vi "notification_option.vi"(11 "your_email":string) -> (1 "pick_up_code":string, 2 "go_to_the_address":string, 3 "to_receive":string)   [LabVIEW 2023]
uses:
  <vilib>/Utility/file.llb/Read Delimited Spreadsheet (string).vi
  Global 1.vi
panel:
  out "substring":string
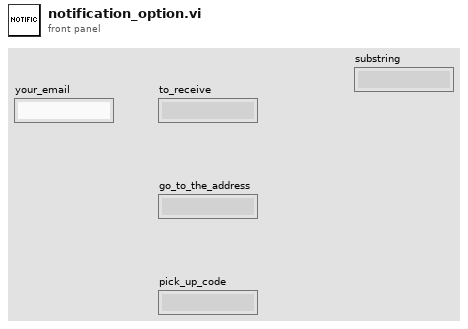
[diagram p1: front panel]
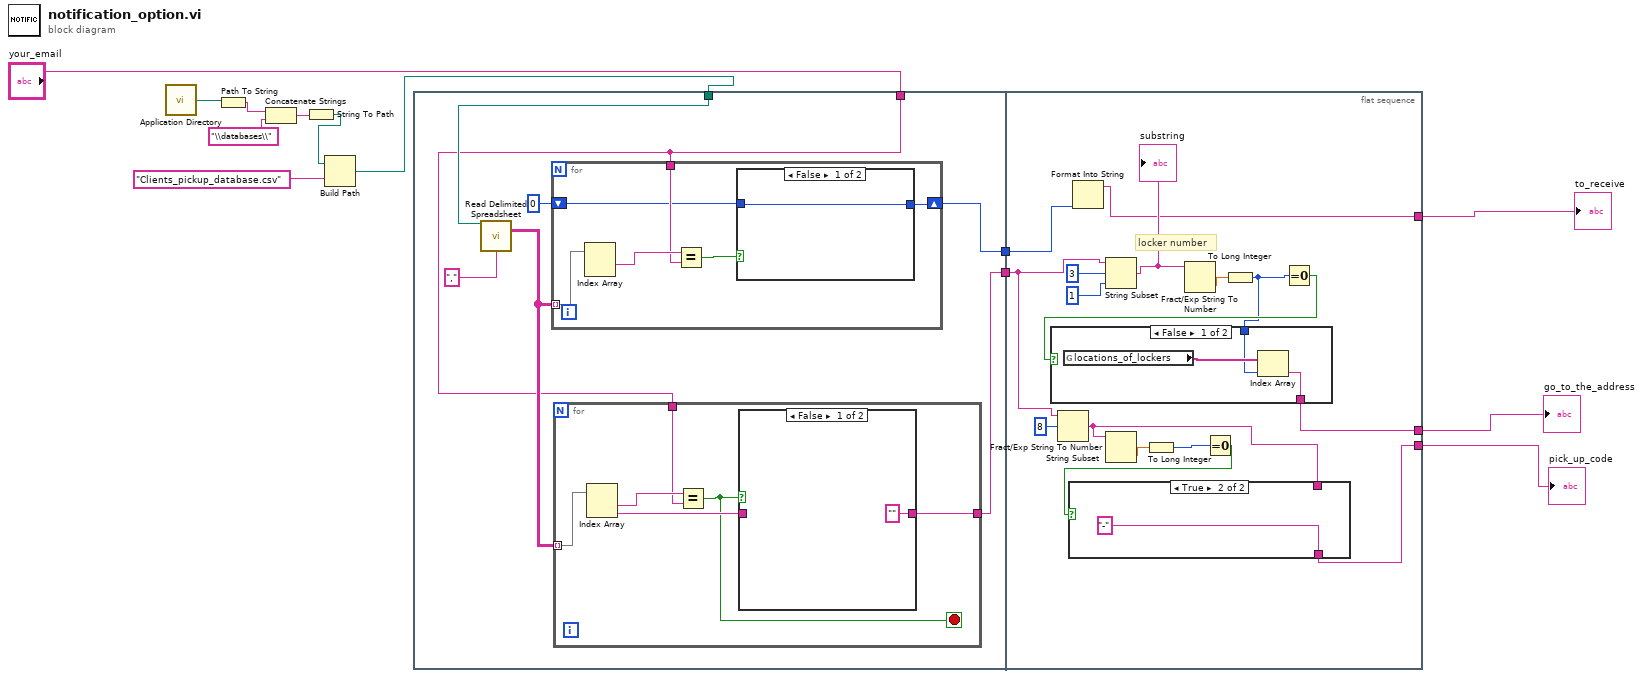
[diagram p0: block diagram]
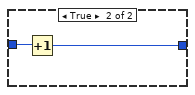
[diagram p3: hidden frame]
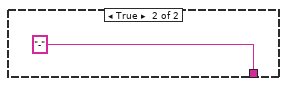
[diagram p5: hidden frame]
diagram:
  n1 = call <vilib>:"Application Directory.vi"() -> ("Application Directory"=w5:path)
  n2 = Path To String(path=w5) -> (string=w6:string)
  n3 = Concatenate Strings(w6, "\\databases\\") -> (w8:string)
  n4 = String To Path(string=w8) -> (path=w9:path)
  n5 = Build Path(base path=w9, name or relative path="Clients_pickup_database.csv") -> (appended path=w10:path)
  n6 = flat-sequence {
    tunnel: w10 -> [w19]
    tunnel: [w14] -> w3
    tunnel: [w17] -> w2
    tunnel: "your_email" -> [w15]
    tunnel: w3 -> [w45]
    tunnel: w2 -> [w51]
    tunnel: [w44] -> w11
    tunnel: [w39] -> w12
    tunnel: [w43] -> w13
    frame #0 {
      n7 = call-poly <vilib>:"Read Delimited Spreadsheet.vi"("file path (dialog if empty)"=w19, "delimiter (\\t)"="," ("delimiter (\\t)")) -> ("all rows"=w16:string[][])  [unwired: 8 in, 5 out]
      n8 = for {
        tunnel: w16 -> [w32] mode=indexing
        tunnel: w15 -> [w33]
        shift-right: [w30] -> w17
        shift-left: 0 -> [w31]
        n9 = Index Array "Index Array"(array=w32) -> (element #1=w34:string)  [unwired: 2 in, 1 out]
        n10 = Equal?(x=w34, y=w33) -> (x = y?=w29:bool)
        n11 = case shown="False" w29 {
          tunnel: w31 -> [w35 w37]
          tunnel: [w35 w36] -> w30
          frame False {
          }
          frame True {
            n12 = Increment(x=w37) -> (x+1=w36:i32)
          }
        }
      }
      n13 = for {
        tunnel: w16 -> [w24] mode=indexing
        tunnel: w15 -> [w25]
        tunnel: [w22] -> w14
        stop <- w21 stop-if-true
        n14 = Index Array "Index Array"(array=w24) -> (element #1=w26:string, element #2=w23:string)  [unwired: 2 in]
        n15 = Equal?(x=w26, y=w25) -> (x = y?=w21:bool)
        n16 = case shown="False" w21 {
          tunnel: w23 -> [_ w28]
          tunnel: ["" ("String") w28] -> w22
          frame False {
          }
          frame True {
          }
        }
      }
    }
    frame #1 {
      # "locker number"
      n17 = String Subset(string=w45, offset (0)=8) -> (substring=w38:string)  [unwired: 1 in]
      n18 = Format Into String(w51) -> (resulting string=w43:string)  [unwired: 3 in, 1 out]
      n19 = String Subset(string=w45, offset (0)=3, length (rest)=1 ("length (rest)")) -> (substring=w50:string)
      "substring" <- w50
      n20 = Fract/Exp String To Number(string=w38) -> (number=w41:dbl)  [unwired: 3 in, 1 out]
      n21 = To Long Integer(number=w41) -> (32bit integer=w42:i32)
      n22 = Fract/Exp String To Number(string=w50) -> (number=w48:dbl)  [unwired: 3 in, 1 out]
      n23 = Equal To 0?(x=w42) -> (x = 0?=w40:bool)
      n24 = case shown="True" w40 {
        tunnel: [w54 "-" ("to_receive 2")] -> w39
        tunnel: w38 -> [w54 _]
        frame False {
        }
        frame True {
        }
      }
      n25 = To Long Integer(number=w48) -> (32bit integer=w47:i32)
      n26 = Equal To 0?(x=w47) -> (x = 0?=w49:bool)
      n27 = case shown="False" w49 {
        tunnel: [w56 "-" ("to_receive 2")] -> w44
        tunnel: w47 -> [w57 _]
        frame False {
          n28 = global read "Global 1.vi" "locations_of_lockers"() -> (w58:string[])
          n29 = Index Array(array=w58, index=w57) -> (element=w56:string)
        }
        frame True {
        }
      }
    }
  }
  "to_receive" <- w13
  "pick_up_code" <- w12
  "go_to_the_address" <- w11
